vi "TekSetup.vi"() -> ()   [LabVIEW 2022 SP3]
panel:
  out "YOffset":dbl
  out "XZero":dbl
  out "YZero":dbl
  out "YMult":dbl
  out "XMult":dbl
  out "s/div":dbl
  out "V/div":dbl
  out "array":string[](array[string])
  out "Scope":cluster{dbl, dbl, dbl[]}(graph)
  in  "write buffer 2":string="DAT:WID?"
  in  "write buffer":string="wavfrm?"
  out "read buffer":string
  in  "VISA resource name":refnum<visa-resource-name>
  # "data?\n:DATA:ENCDG ASCII;DESTINATION REFA;SOURCE CH1;START 1;STOP 2500;WIDTH 1"
  # "*IDN? - returns scope info\ndata:source ch1 - no reply\ndata:width - should be 1 byte\ndata:encdg? - should be ASCII\ndata:source? - ch1\nch1? - all the info on the scale etc\nhor:main:scale? - time res\nhead 0 - turn off headers so only numbers are returned\nset? - returns all settings\ntrigger:main:mode auto - or normal\ntrigger:state? - shoudl return armed or ready (or auto)\nwavfrm? - returns settings and curve - very nice\n*OPC? - waits until everything is done?"
  # "set?\n:HEADER 1;:VERBOSE 1;:DATA:ENCDG ASCII;DESTINATION REFA;SOURCE CH1;START 1;STOP 2500;WIDTH 1;:LOCK NONE;:DISPLAY:FORMAT YT;STYLE VECTORS;PERSISTENCE 0;BACKLIGHT 100;:ACQUIRE:MODE SAMPLE;NUMAVG 16;STATE 1;STOPAFTER RUNSTOP;:CH1:PROBE 1.0E1;CURRENTPROBE 1.0E1;SCALE 2.0E0;POSITION 0.0E0;COUPLING DC;BANDWIDTH OFF;INVERT OFF;YUNIT \"V\";:CH2:PROBE 1.0E1;CURRENTPROBE 1.0E1;SCALE 2.0E0;POSITION 0.0E0;COUPLING DC;BANDWIDTH OFF;INVERT OFF;YUNIT \"V\";:HORIZONTAL:MAIN:SCALE 5.0E-4;POSITION 0.0E0;:TRIGGER:MAIN:MODE AUTO;TYPE EDGE;HOLDOFF:VALUE 5.0E-7;:TRIGGER:MAIN:EDGE:SOURCE CH1;COUPLING DC;SLOPE RISE;:TRIGGER:MAIN:VIDEO:SOURCE CH1;SYNC LINE;POLARITY NORMAL;LINE 1;STANDARD NTSC;:TRIGGER:MAIN:PULSE:SOURCE CH1;WIDTH:POLARITY POSITIVE;WHEN EQUAL;WIDTH 1.0E-3;:TRIGGER:MAIN:LEVEL 0.0E0;:SELECT:FFT 0;CH1 1;CH2 0;MATH 0;REFA 0;REFB 0;:CURSOR:FUNCTION OFF;SELECT:SOURCE CH1;:CURSOR:VBARS:UNITS SECONDS;POSITION1 -2.0E-3;POSITION2 2.0E-3;:CURSOR:HBARS:POSITION1 6.4E0;POSITION2 -6.4E0;:MEASUREMENT:MEAS1:TYPE NO"
  # "trigger?\n:TRIGGER:MAIN:MODE AUTO;TYPE EDGE;HOLDOFF:VALUE 5.0E-7;:TRIGGER:MAIN:EDGE:SOURCE CH1;COUPLING DC;SLOPE RISE;:TRIGGER:MAIN:VIDEO:SOURCE CH1;SYNC LINE;POLARITY NORMAL;LINE 1;STANDARD NTSC;:TRIGGER:MAIN:PULSE:SOURCE CH1;WIDTH:POLARITY POSITIVE;WHEN EQUAL;WIDTH 1.0E-3;:TRIGGER:MAIN:LEVEL 0.0E0"
  # "wavfrm?\n:WFMPRE:BYT_NR 1;BIT_NR 8;ENCDG ASC;BN_FMT RP;BYT_OR MSB;NR_PT 2500;WFID \"Ch1, DC coupling, 2.0E0 V/div, 5.0E-4 s/div, 2500 points, Sample mode\";PT_FMT Y;XINCR 2.0E-6;PT_OFF 0;XZERO -2.5E-3;XUNIT \"s\";YMULT 8.0E-2;YZERO 0.0E0;YOFF 0.0E0;YUNIT \"Volts\";:CURVE 0,0,0,0,1,0,0,0,0,1,0,0,0,1,1,0,0,0,0,0,0,0,0,0,0,0,0,0,0,1,0,1,0,0,0,0,0,0,0,0,1,0,0,0,0,0,0,0,0,0,0,0,0,0,0,1,0,0,0,1,0,0,0,0,0,0,0,0,0,1,0,0,0,0,0,0,0,0,0,1,0,0,0,0,0,0,0,1,0,0,0,0,0,0,0,1,0,0,0,0,0,0,1,0,0,0,0,0,0,0,0,0,0,0,0,0,1,0,0,0,1,1,1,1,0,0,0,1,0,0,0,0,0,1,0,0,1,1,0,0,1,0,0,0,0,0,0,0,0,1,0,0,0,0,0,0,1,0,0,1,0,1,0,0,0,0,0,1,0,0,0,0,0,0,0,0,0,0,1,0,1,0,1,0,0,0,0,0,0,0,0,0,0,0,0,0,0,1,0,0,0,0,1,0,0,0,1,0,0,1,0,0,0,1,0,1,0,1,0,0,0,0,0,0,0,0,1,0,1,0,0,0,0,0,0,1,0,1,0,0,0,0,0,0,0,0,0,0,0,0,1,0,1,0,0,0,1,1,1,0,0,0,0,0,1,1,0,0,1,0,1,1,0,0,0,1,1,0,0,0,0,-1,1,0,0,1,0,0,0,0,0,0,1,0,1,0,1,0,0,0,0,0,0,0,0,1,1,0,0,0,0,0,0,0,0,0,0,1,1,0,0,0,0,0,0,0,0,0,0,0,1,0,0,0,0,0,0,0,0,0,1,1,0,1,0,0,0,0,0,0,0,1,0,1,0,0,0,1,0,1,0,0,0,0,0,0,1,0,0,1,0,"
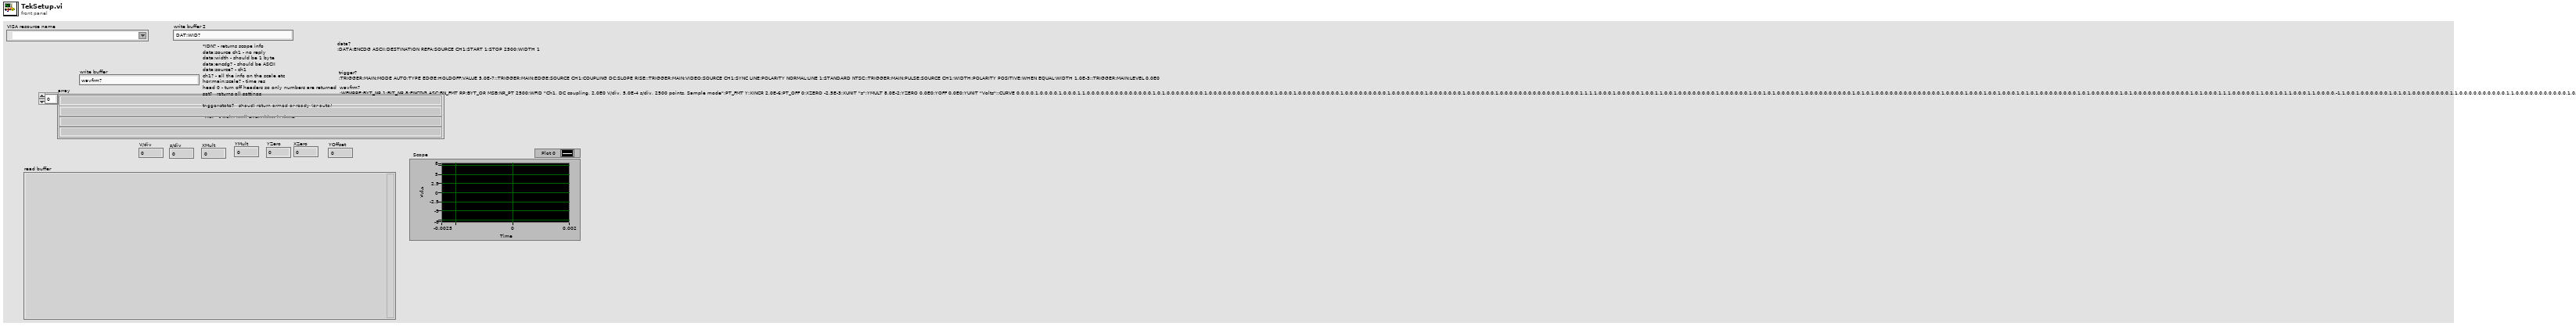
[diagram p1: front panel]
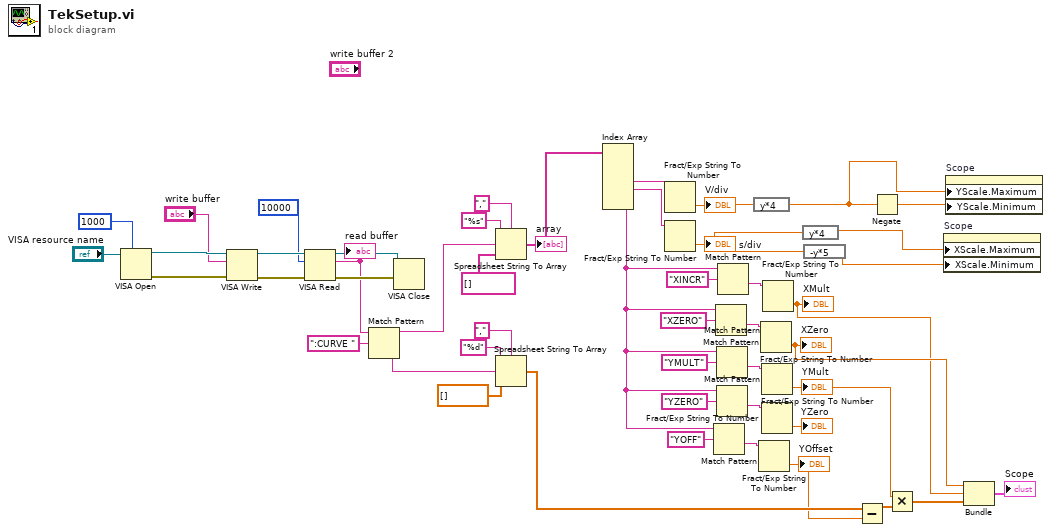
[diagram p0: block diagram]
diagram:
  n1 = VISA Open(timeout (0)=u32 1000 ("VISA Open timeout (0)"), VISA resource name="VISA resource name") -> (VISA resource name=w49:refnum<visa-resource-name>, error out=w47:errorcluster)  [unwired: 3 in]
  n2 = VISA Write(VISA resource name=w49, write buffer="write buffer", error in (no error)=w47) -> (VISA resource name out=w45:refnum<visa-resource-name>, error out=w46:errorcluster)  [unwired: 1 out]
  n3 = VISA Read(VISA resource name=w45, byte count=u32 10000, error in (no error)=w46) -> (VISA resource name out=w42:refnum<visa-resource-name>, read buffer=w40:string, error out=w41:errorcluster)  [unwired: 1 out]
  "read buffer" <- w40
  n4 = Match Pattern(string=w40, regular expression=":CURVE ") -> (before substring=w32:string, after substring=w35:string)  [unwired: 1 in, 2 out]
  n5 = VISA Close(VISA resource name=w42, error in (no error)=w41) -> ()  [unwired: 1 out]
  n6 = Spreadsheet String To Array(delimiter (Tab)=",", format string="%s", spreadsheet string=w32, array type (2D Dbl)=string[] []) -> (array=w30:string[])
  "array" <- w30
  n7 = Spreadsheet String To Array(delimiter (Tab)=",", format string="%d", spreadsheet string=w35, array type (2D Dbl)=dbl[] []) -> (array=w19:dbl[])
  n8 = Index Array(array=w30) -> (element #3=w29:string, element #4=w28:string, element #6=w9:string)  [unwired: 6 in, 3 out]
  n9 = Fract/Exp String To Number(string=w29) -> (number=w7:dbl)  [unwired: 3 in, 1 out]
  "V/div" <- w7
  n10 = Fract/Exp String To Number(string=w28) -> (number=w3:dbl)  [unwired: 3 in, 1 out]
  "s/div" <- w3
  n11 = Match Pattern(string=w9, regular expression="YOFF") -> (after substring=w11:string)  [unwired: 1 in, 3 out]
  n12 = Match Pattern(string=w9, regular expression="XZERO") -> (after substring=w21:string)  [unwired: 1 in, 3 out]
  n13 = Match Pattern(string=w9, regular expression="YMULT") -> (after substring=w25:string)  [unwired: 1 in, 3 out]
  n14 = Match Pattern(string=w9, regular expression="YZERO") -> (after substring=w22:string)  [unwired: 1 in, 3 out]
  n15 = Match Pattern(string=w9, regular expression="XINCR") -> (after substring=w26:string)  [unwired: 1 in, 3 out]
  n16 = expression code="y*4"(w7) -> (w6:dbl)
  n17 = Fract/Exp String To Number(string=w11) -> (number=w8:dbl)  [unwired: 3 in, 1 out]
  "YOffset" <- w8
  n18 = Fract/Exp String To Number(string=w21) -> (number=w15:dbl)  [unwired: 3 in, 1 out]
  "XZero" <- w15
  n19 = Fract/Exp String To Number(string=w25) -> (number=w16:dbl)  [unwired: 3 in, 1 out]
  "YMult" <- w16
  n20 = Fract/Exp String To Number(string=w22) -> (number=→"YZero":dbl)  [unwired: 3 in, 1 out]
  n21 = Fract/Exp String To Number(string=w26) -> (number=w14:dbl)  [unwired: 3 in, 1 out]
  "XMult" <- w14
  n22 = expression code="y*4"(w3) -> (w4:dbl)
  n23 = expression code="-y*5"(w3) -> (w2:dbl)
  n24 = Subtract(x=w19, y=w8) -> (x-y=w17:dbl[])
  n25 = Negate(x=w6) -> (-x=w5:dbl)
  n26 = Multiply(x=w16, y=w17) -> (x*y=w13:dbl[])
  n27 = property on="Scope" class="WFGraph (strict)"("XScale.Maximum"=w4, "XScale.Minimum"=w2) -> ()  [unwired: 2 in, 2 out]
  n28 = property on="Scope" class="WFGraph (strict)"("YScale.Maximum"=w6, "YScale.Minimum"=w5) -> ()  [unwired: 2 in, 2 out]
  n29 = Bundle(w15, w14, w13) -> (→"Scope":cluster{dbl, dbl, dbl[]})  [unwired: 1 in]
